vi "DigitalOut.vi"(8 "error in (no error)":errorcluster, 9 "Existing Obj Name":string, 10 "pin":string, 11 "mbed_LVLibrary.lvlib:mbed.lvclass":refnum<class "mbed.lvclass">) -> (0 "error out":errorcluster, 1 "Assigned Name":string, 3 "DigitalOut.lvclass":refnum<class "DigitalOut.lvclass">)   [LabVIEW 2011, in "mbed_LVLibrary.lvlib" / "DigitalOut.lvclass"]
doc: "This is the DigitalOut constructor. It takes either the pin number as a string (eg \"p21\" or \"LED1\") or the name of an existing DigitalOut object on mbed. If a pin number is given the object is created using RPC.\nThe Assigned name output is the name given to the object by the RPC handler. It is only of interest for checking correct operation or for manually entering RPC commands for that object."
uses:
  DigitalOut.lvclass
  Transport Mechanisms/mbed/mbed.lvclass
  DigitalOut.lvclass/DigitalOut.ctl
  <vilib>/regexp/Match Regular Expression.xnode
panel:
  in  "DigitalOut.lvclass 2":refnum<class "DigitalOut.lvclass">
  # "This is the constructor for a new Digital Out"
  # "Takes an mbed class (which contains the transport method)\n and puts it as a memeber of the Digital Out class\nIt also either ties an existing instance on mbed or creates one"
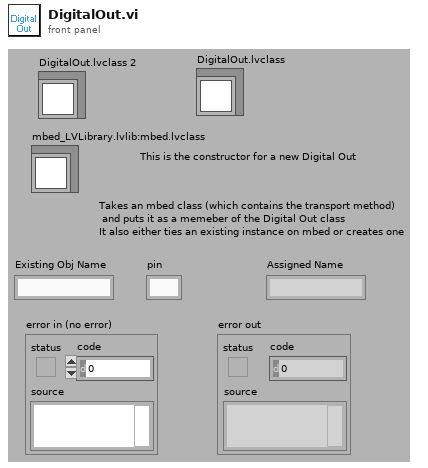
[diagram p1: front panel]
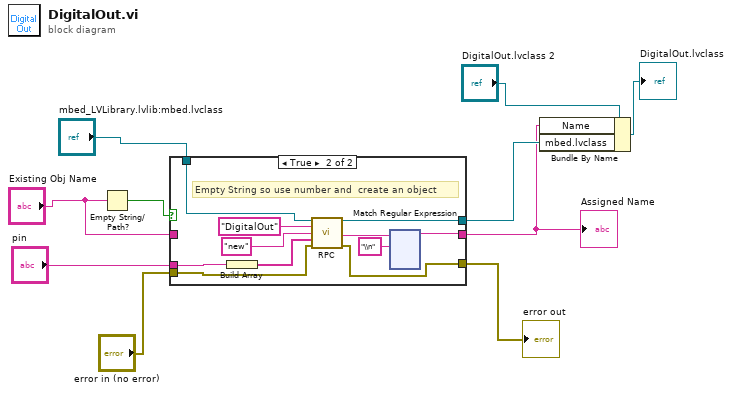
[diagram p0: block diagram]
diagram:
  n1 = Empty String/Path?(string/path="Existing Obj Name") -> (empty?=w5:bool)
  n2 = case shown="True" w5 {
    tunnel: "Existing Obj Name" -> [w13 _]
    tunnel: [w13 w20] -> w6
    tunnel: "mbed_LVLibrary.lvlib:mbed.lvclass" -> [w12 w24]
    tunnel: [w12 w21] -> w7
    tunnel: "pin" -> [_ w17]
    tunnel: "error in (no error)" -> [w11 w15]
    tunnel: [w11 w14] -> w2
    frame False {
      # "String present so just set the class name"
    }
    frame True {
      # "Empty String so use number and  create an object"
      n3 = Build Array(w17) -> (w16:string[])
      n4 = call-dynamic "RPC.vi"("mbed in"=w24, "Name"="DigitalOut", "method"="new", "Args"=w16, "error in (no error)"=w15) -> ("mbed out"=w21:refnum<class "mbed.lvclass">, "RPC Result"=w19:string, "error out"=w14:errorcluster)  [unwired: 8 in]
      n5 = xnode "Match Regular Expression"("input string"=w19, "regular expression"="\\n") -> ("before match"=w20:string)  [unwired: 4 in, 4 out]
    }
  }
  "Assigned Name" <- w6
  "error out" <- w2
  n6 = Bundle By Name(cluster="DigitalOut.lvclass 2", "Name"=w6, "mbed.lvclass"=w7) -> (→"DigitalOut.lvclass":refnum<class "DigitalOut.lvclass">)
